vi "upload.initiate_multipart_upload.vi"(8 "error in":errorcluster, 10 "File Path":path, 11 "Nominal Client in":refnum<class "Nominal Client.lvclass">) -> (0 "error out":errorcluster, 2 "Multipart Upload":refnum<class "Multipart Upload.lvclass">, 3 "Nominal Client out":refnum<class "Nominal Client.lvclass">)   [LabVIEW 2020, in "Multipart Upload.lvclass"]
doc: "Initiates a multipart upload to S3. Does not directly upload any parts, but returns an uploadId used to upload parts."
uses:
  Multipart Upload.lvclass
  Nominal Client/Nominal Client.lvclass
  Nominal Client/Nominal Client.lvclass/Nominal Client.ctl
  nominal types/workspace/workspace.lvclass/workspace.ctl
  Multipart Upload.lvclass/Multipart Upload.ctl
  8b3dcdab-c30a-41f7-882b-0fd92512159b.vi
  Nominal Client/workspace.get.vi
  <vilib>/JDP Science/JSONtext/Merge into Object.vi
  Nominal Client/workspace.add_to_payload.vi/88650e10-de3e-481c-85db-71cb0fdf4485.vi
  nominal types/workspace/rid.get.vi
  <vilib>/Utility/libraryn.llb/Get File Extension.vi
  <vilib>/JDP Science/JSONtext/Variant to JSON Text.vi
  <vilib>/JDP Science/JSONtext/Get all Object Items.vi
  <vilib>/JDP Science/JSONtext/Set Multiple Object Items.vi
  <vilib>/JDP Science/JSONtext/JSON text to Variant.vi
  <vilib>/JDP Science/JSONtext/LVClass Serializer/JSONtext LVClass Serializer.lvclass
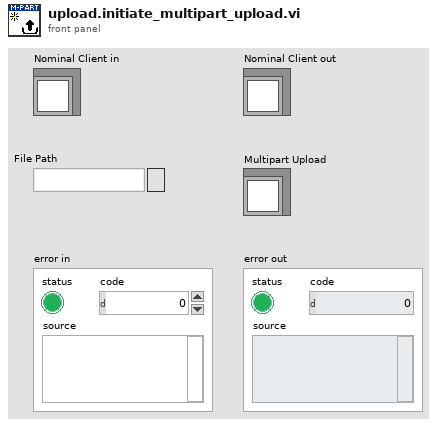
[diagram p1: front panel]
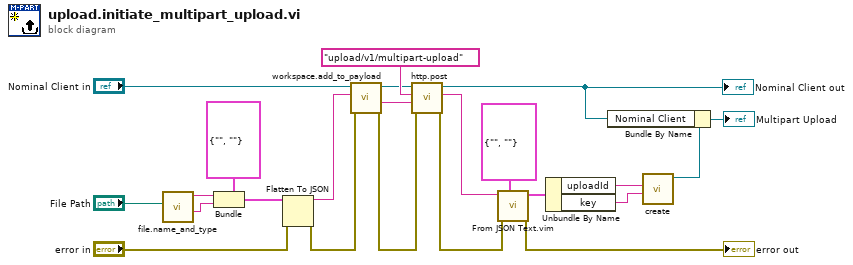
[diagram p0: block diagram]
diagram:
  n1 = call "file.name_and_type.vi"("File Path"="File Path") -> ("File Type"=w15:string, "File Name"=w16:string)  [unwired: 8 in, 1 out]
  n2 = Bundle(cluster=cluster{"filename":string, "filetype":string} {"filename"="", "filetype"=""}, "filename"=w16, "filetype"=w15) -> (w22:cluster{"filename":string, "filetype":string})
  n3 = Flatten To JSON(anything=w22, error in (no error)="error in") -> (JSON string=w4:string, 11:w2:errorcluster)  [unwired: 1 in]
  n4 = call "workspace.add_to_payload.vi"("error in"=w2, "JSON payload in"=w4, "Nominal Client in"="Nominal Client in") -> ("error out"=w3:errorcluster, "JSON payload out"=w1:string, "Nominal Client out"=w5:refnum<class "Nominal Client.lvclass">)  [unwired: 6 in]
  n5 = call "http.post.vi"("error in"=w3, "Request body"=w1, "Path"="upload/v1/multipart-upload", "Nominal Client in"=w5) -> ("error out"=w14:errorcluster, "Response"=w18:string, "Nominal Client out"=w8:refnum<class "Nominal Client.lvclass">)  [unwired: 5 in]
  "Nominal Client out" <- w8
  n6 = call "From JSON Text.vim"("Data Type and Default Value"=cluster{"uploadId":string, "key":string} {"uploadId"="", "key"=""}, "error in (no error)"=w14, "JSON"=w18) -> ("error out"=→"error out":errorcluster, "Data out"=w13:cluster{"uploadId":string, "key":string})  [unwired: 7 in]
  n7 = Unbundle By Name(w13) -> ("uploadId"=w11:string, "key"=w10:string)
  n8 = call "create.vi"("Key"=w10, "Upload ID"=w11) -> ("Nominal Client MultiPart Upload"=w9:refnum<class "Multipart Upload.lvclass">)  [unwired: 8 in, 1 out]
  n9 = Bundle By Name(cluster=w9, "Nominal Client"=w8) -> (→"Multipart Upload":refnum<class "Multipart Upload.lvclass">)
